vi "SetErr_ParamNotFound.vi"(10 "param":string, 11 "_ConfigClass_INI.lvlib:_ConfigClass_INI_IN":refnum<class "_ConfigClass_INI.lvclass">) -> (0 "error_OUT":errorcluster, 3 "_ConfigClass_INI.lvlib:_ConfigClass_INI_OUT":refnum<class "_ConfigClass_INI.lvclass">)   [LabVIEW 2019, in "_ConfigClass_INI.lvlib" / "_ConfigClass_INI.lvclass"]
uses:
  _ConfigClass_INI.lvclass
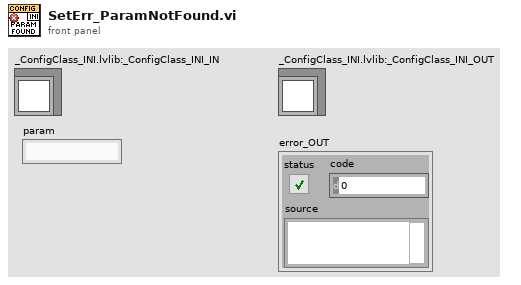
[diagram p1: front panel]
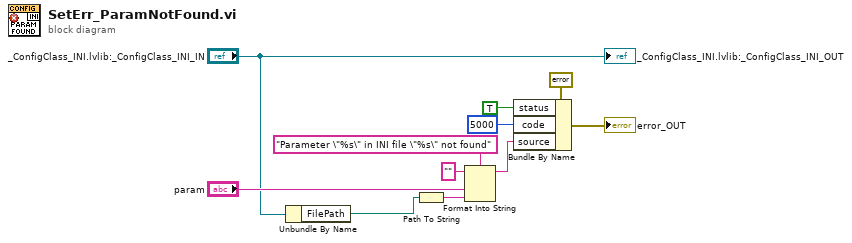
[diagram p0: block diagram]
diagram:
  n1 = Unbundle By Name("_ConfigClass_INI.lvlib:_ConfigClass_INI_IN") -> ("FilePath"=w2:path)
  n2 = Path To String(path=w2) -> (string=w8:string)
  n3 = Format Into String(format string="Parameter \"%s\" in INI file \"%s\" not found" ("source"), initial string="", "param", w8) -> (resulting string=w9:string)  [unwired: 1 in, 1 out]
  n4 = Bundle By Name(cluster=errorcluster {"status"=FALSE, "code"=0, "source"=""} ("input cluster"), "status"=TRUE, "code"=5000, "source"=w9) -> (→"error_OUT":errorcluster)
  "_ConfigClass_INI.lvlib:_ConfigClass_INI_OUT" <- "_ConfigClass_INI.lvlib:_ConfigClass_INI_IN"
